vi "Write Response Queue.vi"(8 "error in (no error)":errorcluster, 10 "RESP3 Value in":variant, 11 "reponse queue":refnum<queue>) -> (0 "error out":errorcluster)   [LabVIEW 2019, in "Test Redis Client for LabVIEW.lvlib"]
uses:
  Test Redis Client for LabVIEW.lvlib
  RESP3 for LabVIEW/RESP3/RESP3.lvlib
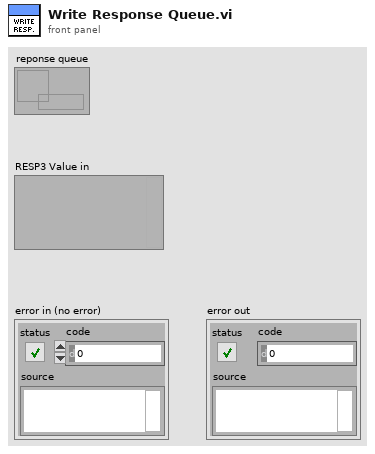
[diagram p1: front panel]
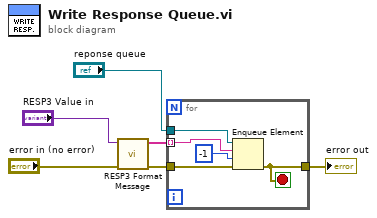
[diagram p0: block diagram]
diagram:
  n1 = call "RESP3 Format Message.vi"("error in (no error)"="error in (no error)", "RESP3 Value"="RESP3 Value in") -> ("error out"=w2:errorcluster, "messages"=w4:string[])  [unwired: 8 in]
  n2 = for {
    tunnel: "reponse queue" -> [w11]
    tunnel: w4 -> [w10] mode=indexing
    tunnel: w2 -> [w8]
    tunnel: [w7] -> w1
    stop <- w7 stop-if-true
    n3 = Enqueue Element(queue=w11, element=w10, timeout in ms (-1)=-1, error in (no error)=w8) -> (error out=w7:errorcluster)  [unwired: 2 out]
  }
  "error out" <- w1
